vi "Shooter Controller.vi"(8 "error in":errorcluster) -> ()   [LabVIEW 2020]
doc: "This VI executes continuously carrying out the current operation and responding to updates or new operations. It will often contain the timing or control code that is difficult to place directly in TeleOp. This VI generally opens all sensors and motors and isolates the rest of the robot code from knowing how the operations are carried out."
uses:
  <vilib>/Rock Robotics/WPI/Framework/Completion Status.ctl
  Shooter Setpoints.ctl
  Shooter Operations.ctl
  <vilib>/Rock Robotics/Network Tables/NT Write Boolean.vi
panel:
  in  "Output 2":dbl=-0.6 format="%#_13g"
  in  "Output":dbl=-0.6 format="%#_13g"
  in  "Interactive Values":T1
  out "Current\nCmd":string
  in  "Buttons":cluster{"Execute Cmd":bool, "Abort Cmd":bool}
  out "Command Timing":cluster{"Start Time (ms)":u32, "Iterations":i32}
  out "Status":T3
  # "Tip: It may be helpful to observe inputs and sensor values.\nYou may also want to display tuning or debugging controls."
  # "Interactive Command: You may fill in the settings for a command\nand schedule it with the Execute button. You can observe and abort\nany command while fine tuning the code for the controller."
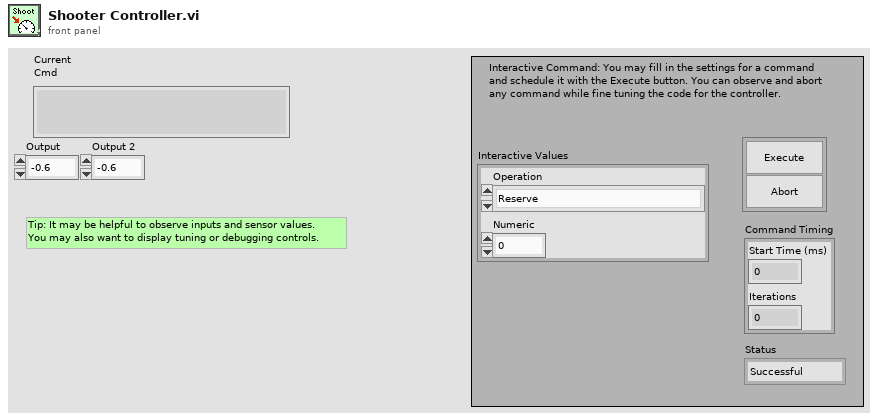
[diagram p1: front panel]
types:
  T1 = typedef "Shooter Setpoints.ctl" = cluster{"Operation":T2, "Numeric":dbl}
  T2 = typedef "Shooter Operations.ctl" = enum16{"Reserve", "Read Current", "Immediate", "Shoot"}
  T3 = typedef "Completion Status.ctl" = enum16{"Successful", "Aborted", "Incomplete"}
  T4 = typedef "Command Status Info.ctl" = cluster{"Name":string, "Status":T3, "notifier out":T5}
  T5 = typedef "Completion Notifier.ctl" = refnum<notifier>
  T6 = cluster{"Current Command":T1, "Command Timing":cluster{"Start Time (ms)":u32, "Iterations":i32}, "Command Arguments":cluster{"Command Info":T4, "Description":string, "Default Command":T1, "queue out":refnum<queue>, "Subsystem Name":string}}
  T7 = typedef "WPI_MotorControlDeviceRef.ctl" = cluster{"DeviceStatus":errorcluster, "Type":T8, "PWM":cluster{"PWM Channel":T9, "DeadBand":T10}, "CAN":cluster{"Device Number":u8, "SetOutput VI Ref":variant, "GetOutput VI Ref":variant, "Enable VI Ref":variant, "Disable VI Ref":variant, "Data":variant}, "Invert":bool, "DIO PWM":cluster{"PWM \"Enable\" Channel":T9, "DIOChannel":T11, "PWM Rate":dbl}}
  T8 = typedef "WPI_MotorControlType.ctl" = enum16{"PWM", "CAN", "DIO PWM"}
  T9 = typedef "FPGA_DIOPWMChannel.ctl" = enum8{"PWM 0", "PWM 1", "PWM 2", "PWM 3", "PWM 4", "PWM 5", "PWM 6", "PWM 7", "PWM 8", "PWM 9", "PWM MXP 0", "PWM MXP 1", "PWM MXP 2", "PWM MXP 3", "PWM MXP 4", "PWM MXP 5", "PWM MXP 6", "PWM MXP 7", "PWM MXP 8", "PWM MXP 9", "Invalid"}
  T10 = typedef "WPI_PWMDeadband.ctl" = cluster{"Name":string, "maxPositivePwm":i32, "minPositivePwm":i32, "centerPwm":i32, "maxNegativePwm":i32, "minNegativePwm":i32, "angularRange":u16}
  T11 = typedef "FPGA_DIOChannel.ctl" = enum8{"DIO 0", "DIO 1", "DIO 2", "DIO 3", "DIO 4", "DIO 5", "DIO 6", "DIO 7", "DIO 8", "DIO 9", "DIO MXP 0", "DIO MXP 1", "DIO MXP 2", "DIO MXP 3", "DIO MXP 4", "DIO MXP 5", "DIO MXP 6", "DIO MXP 7", "DIO MXP 8", "DIO MXP 9", "DIO MXP 10", "DIO MXP 11", "DIO MXP 12", "DIO MXP 13", "DIO MXP 14", "DIO MXP 15", "SPI Port CS1", "SPI Port CS2", "SPI Port CS3", "SPI Port MISO", "SPI Port MOSI", "Invalid"}
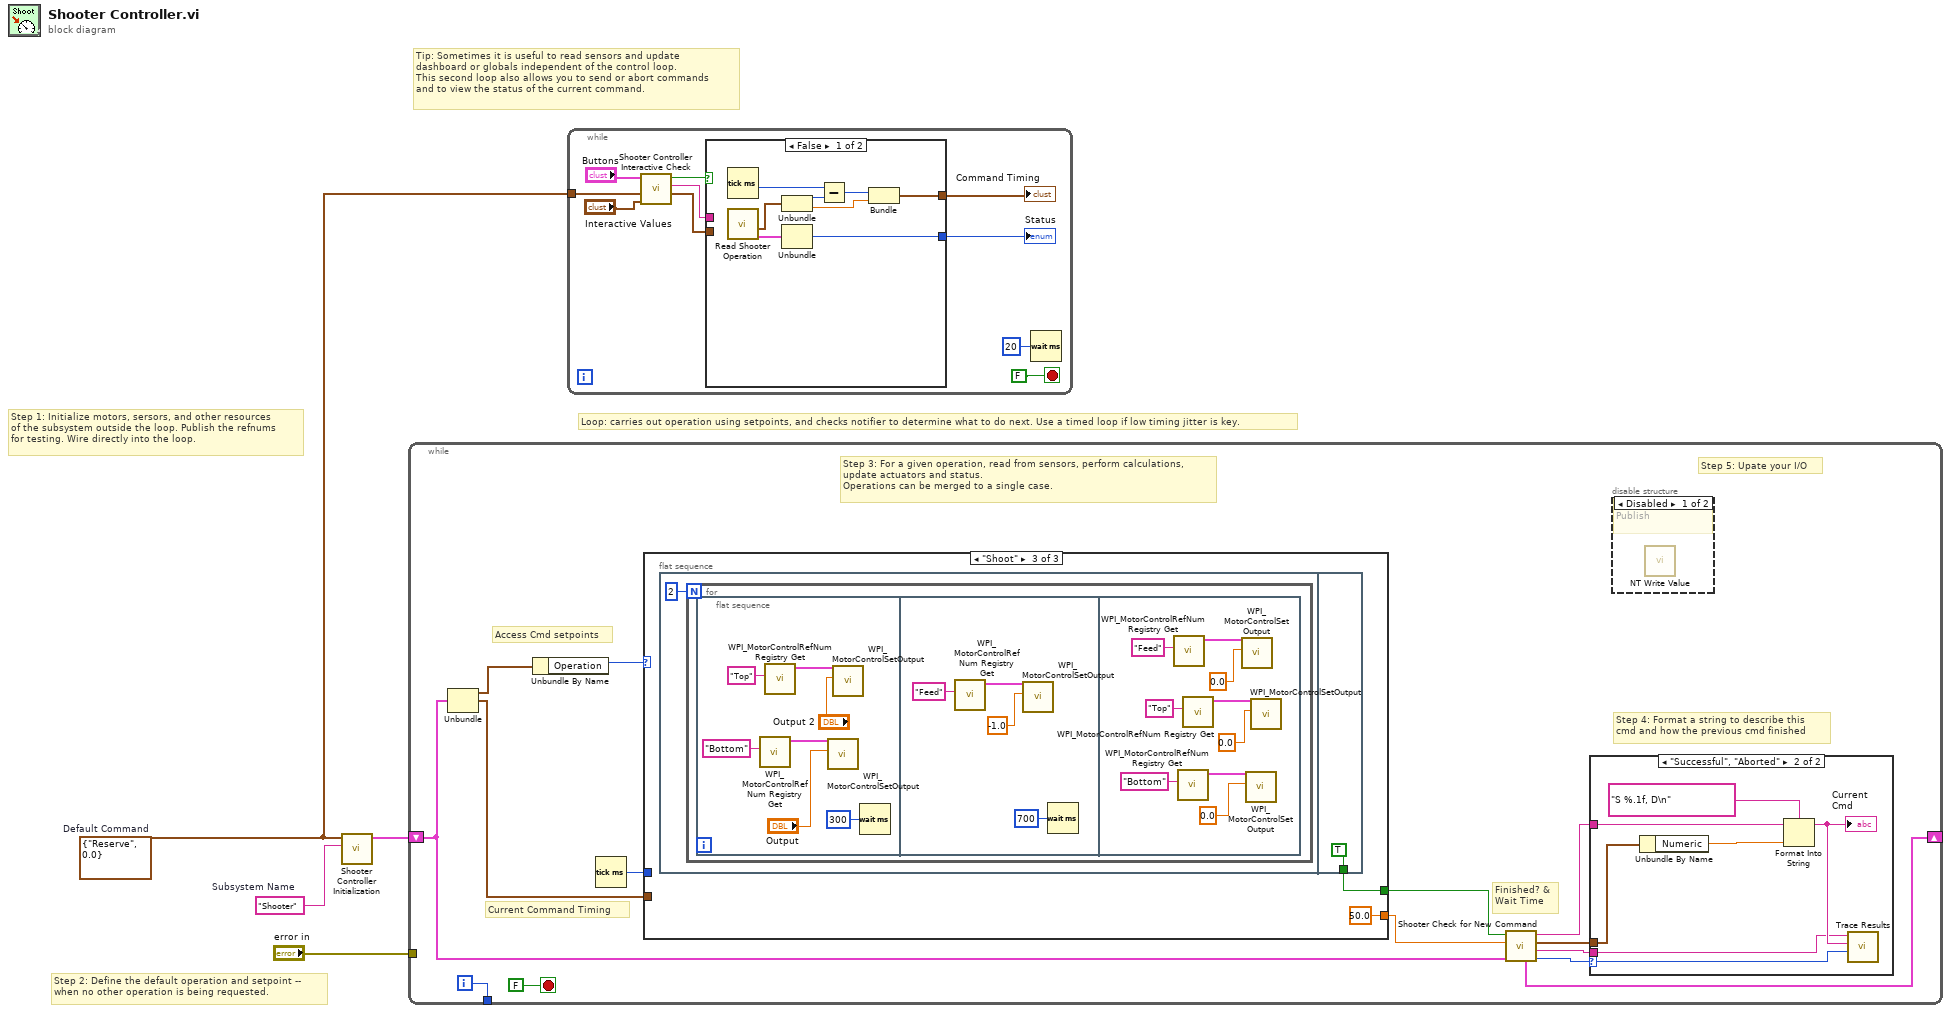
[diagram p0: block diagram]
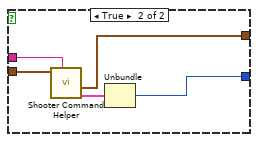
[diagram p2: hidden frame]
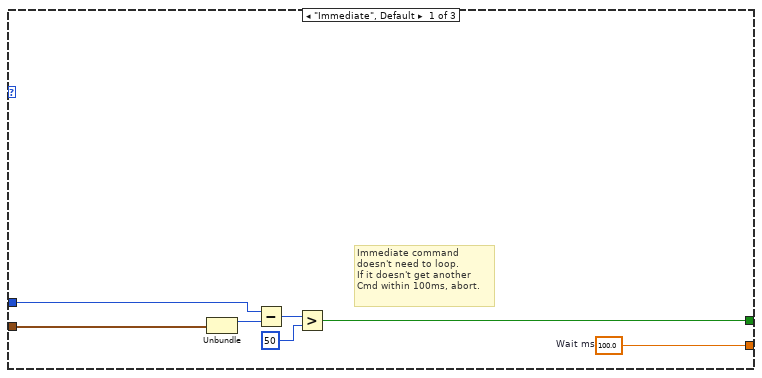
[diagram p5: hidden frame]
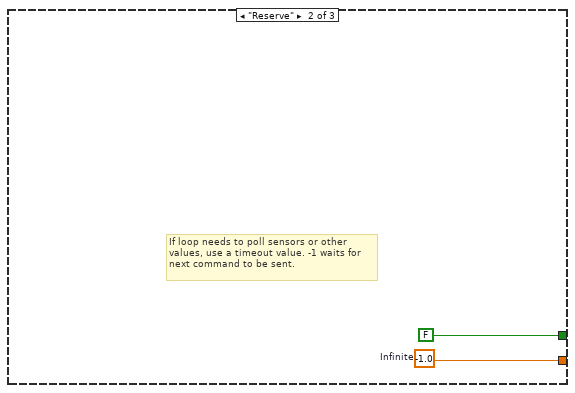
[diagram p6: hidden frame]
diagram:
  w1 = T1 {"Operation"=enum."Reserve", "Numeric"=0.0}  # Default Command
  w2 = "Shooter"  # Subsystem Name
  # "Tip: Sometimes it is useful to read sensors and update\ndashboard or globals independent of the control loop.\nThis second loop also allows you to send or abort commands\nand to view the status of the current command."
  # "Step 2: Define the default operation and setpoint --\nwhen no other operation is being requested."
  # "Step 1: Initialize motors, sersors, and other resources\nof the subsystem outside the loop. Publish the refnums\nfor testing. Wire directly into the loop."
  # "Loop: carries out operation using setpoints, and checks notifier to determine what to do next. Use a timed loop if low timing jitter is key."
  n1 = call "Shooter Controller Initialization.vi"("Subsystem Name"=w2, "Default Command"=w1) -> ("Current Command"=w3:T6)  [unwired: 9 in]
  n2 = while {
    shift-right: [w12] -> _
    shift-left: w3 -> [w5]
    tunnel: [w17] -> _
    tunnel: "error in" -> [_]
    i -> [w17]
    stop <- FALSE stop-if-true
    # "Step 5: Upate your I/O"
    # "Step 4: Format a string to describe this\ncmd and how the previous cmd finished"
    # "Current Command Timing"
    # "Access Cmd setpoints"
    # "Finished? &\nWait Time"
    # "Step 3: For a given operation, read from sensors, perform calculations,\nupdate actuators and status.\nOperations can be merged to a single case."
    n3 = Unbundle(w5) -> ("Current Command"=w16:T1, "Command Timing"=w13:cluster{"Start Time (ms)":u32, "Iterations":i32})  [unwired: 1 out]
    n4 = Unbundle By Name(w16) -> ("Operation"=w15:T2)
    n5 = Tick Count (ms)() -> (millisecond timer value=w14:u32)
    n6 = case shown="\"Shoot\"" w15 {
      tunnel: [w32 w34 50.0 ("Infinite")] -> w10
      tunnel: [w26 FALSE ("ignore previous (F)") w35] -> w11
      tunnel: w13 -> [w28 _ _]
      tunnel: w14 -> [w27 _ _]
      frame "Immediate", Default {
        w32 = 100.0  # Wait ms
        # "Immediate command\ndoesn't need to loop.\nIf it doesn't get another\nCmd within 100ms, abort."
        n7 = Unbundle(w28) -> ("Start Time (ms)"=w31:u32)  [unwired: 1 out]
        n8 = Subtract(x=w27, y=w31) -> (x-y=w30:u32)
        n9 = Greater?(x=w30, y=u8 50 ("Left Motor")) -> (0:w26:bool)
      }
      frame "Reserve" {
        w34 = -1.0  # Infinite
        # "If loop needs to poll sensors or other\nvalues, use a timeout value. -1 waits for\nnext command to be sent."
      }
      frame "Shoot" {
        n10 = flat-sequence {
          tunnel: [TRUE ("ignore previous (F)")] -> w35
          frame #0 {
            n11 = for {
              N: 2 -> [_]
              n12 = flat-sequence {
                frame #0 {
                  n13 = call <vilib>:"WPI_MotorControlRefNum Registry Get.vi"("refnum name"="Bottom") -> ("MotorControlDevRef"=w41:T7)  [unwired: 9 in, 1 out]
                  n14 = call <vilib>:"WPI_MotorControlRefNum Registry Get.vi"("refnum name"="Top") -> ("MotorControlDevRef"=w43:T7)  [unwired: 9 in, 1 out]
                  n15 = call <vilib>:"WPI_MotorControlSetOutput.vi"("Output"="Output", "MotorControlDevRef"=w41) -> ()  [unwired: 7 in, 3 out]
                  n16 = call <vilib>:"WPI_MotorControlSetOutput.vi"("Output"="Output 2", "MotorControlDevRef"=w43) -> ()  [unwired: 7 in, 3 out]
                  n17 = Wait (ms)(milliseconds to wait=u32 300) -> ()  [unwired: 1 out]
                }
                frame #1 {
                  n18 = call <vilib>:"WPI_MotorControlRefNum Registry Get.vi"("refnum name"="Feed") -> ("MotorControlDevRef"=w47:T7)  [unwired: 9 in, 1 out]
                  n19 = call <vilib>:"WPI_MotorControlSetOutput.vi"("Output"=-1.0, "MotorControlDevRef"=w47) -> ()  [unwired: 7 in, 3 out]
                  n20 = Wait (ms)(milliseconds to wait=u32 700) -> ()  [unwired: 1 out]
                }
                frame #2 {
                  n21 = call <vilib>:"WPI_MotorControlRefNum Registry Get.vi"("refnum name"="Feed") -> ("MotorControlDevRef"=w56:T7)  [unwired: 9 in, 1 out]
                  n22 = call <vilib>:"WPI_MotorControlRefNum Registry Get.vi"("refnum name"="Bottom") -> ("MotorControlDevRef"=w52:T7)  [unwired: 9 in, 1 out]
                  n23 = call <vilib>:"WPI_MotorControlRefNum Registry Get.vi"("refnum name"="Top") -> ("MotorControlDevRef"=w50:T7)  [unwired: 9 in, 1 out]
                  n24 = call <vilib>:"WPI_MotorControlSetOutput.vi"("Output"=0.0, "MotorControlDevRef"=w56) -> ()  [unwired: 7 in, 3 out]
                  n25 = call <vilib>:"WPI_MotorControlSetOutput.vi"("Output"=0.0, "MotorControlDevRef"=w52) -> ()  [unwired: 7 in, 3 out]
                  n26 = call <vilib>:"WPI_MotorControlSetOutput.vi"("Output"=0.0, "MotorControlDevRef"=w50) -> ()  [unwired: 7 in, 3 out]
                }
              }
            }
          }
          frame #1 {
          }
        }
      }
    }
    n27 = call "Shooter Check for New Command.vi"("Current Command"=w5, "Wait time (ms)"=w10, "Finished?"=w11) -> ("Completion"=w6:T3, "Subsystem Name"=w7:string, "Current Command"=w8:T1, "Initial Trace String"=w9:string, "NextCommand"=w12:T6)  [unwired: 4 in]
    n28 = case shown="\"Successful\", \"Aborted\"" w6 {
      selector: w6 -> [_ w25]
      tunnel: w9 -> [_ w21]
      tunnel: w8 -> [_ w22]
      tunnel: w7 -> [_ w19]
      frame "Incomplete", Default {
        # "Continuing current command"
      }
      frame "Successful", "Aborted" {
        # "Report and setup for next command"
        n29 = Unbundle By Name(w22) -> ("Numeric"=w24:dbl)
        n30 = Format Into String(format string="S %.1f, D\n", initial string=w21, w24) -> (resulting string=w20:string)  [unwired: 1 in, 1 out]
        "Current\nCmd" <- w20
        n31 = call <vilib>:"Trace Results.vi"("Status of previous command"=w25, "Description"=w20, "Subsystem"=w19) -> ()  [unwired: 9 in]
      }
    }
    n32 = disable-structure shown="Disabled" {
      frame Disabled {
        # "Publish"
        n33 = call-poly <vilib>:"NT Write Value.vi"() -> ()  [unwired: 11 in, 1 out]
      }
      frame Enabled {
      }
    }
  }
  n34 = while {
    tunnel: w1 -> [w65]
    stop <- FALSE stop-if-true
    n35 = call "Shooter Controller Interactive Check.vi"("Interactive Command in"="Interactive Values", "Default Command"=w65, "Buttons"="Buttons") -> ("Interactive Command out"=w62:T1, "Trace String"=w63:string, "Schedule"=w64:bool)  [unwired: 6 in]
    n36 = case shown="False" w64 {
      tunnel: [w76 w81] -> w61
      tunnel: w62 -> [_ w79]
      tunnel: [w72 w77] -> w60
      tunnel: w63 -> [_ w80]
      frame False {
        n37 = Tick Count (ms)() -> (millisecond timer value=w71:u32)
        n38 = call "Read Shooter Operation.vi"() -> ("Command Info"=w69:T4, "SubSystem Data"=w70:T1)  [unwired: 9 in, 1 out]
        n39 = Unbundle(w70) -> ("Operation"=w75:T2, "Numeric"=w73:dbl)
        n40 = Unbundle(w69) -> ("Status"=w76:T3)  [unwired: 2 out]
        n41 = Subtract(x=w71, y=w75) -> (x-y=w74:u32)
        n42 = Bundle(w74, "Numeric"=w73) -> (w72:cluster{u32, "Numeric":dbl})  [unwired: 1 in]
      }
      frame True {
        n43 = call "Shooter Command Helper.vi"("Description"=w80, "SubSystem Data"=w79) -> ("Command Info Out"=w78:T4, "Command Timing"=w77:cluster{"Start Time (ms)":u32, "Iterations":i32})  [unwired: 7 in, 1 out]
        n44 = Unbundle(w78) -> ("Status"=w81:T3)  [unwired: 2 out]
      }
    }
    "Status" <- w61
    "Command Timing" <- w60
    n45 = Wait (ms)(milliseconds to wait=u32 20) -> ()  [unwired: 1 out]
  }
